vi "Get AccessType.vi"(8 "error in (no error)":errorcluster, 11 "PDO Mapping in":refnum<class "PDO Mapping.lvclass">) -> (0 "error out":errorcluster, 2 "AccessType":T1, 3 "PDO Mapping out":refnum<class "PDO Mapping.lvclass">)   [LabVIEW 2020, in "CANopen.lvlib" / "PDO Mapping.lvclass"]
uses:
  PDO Mapping.lvclass
  PDO Mapping.lvclass/PDO Mapping.ctl
  Typedefs/Access Type.ctl
  CANopen.lvlib
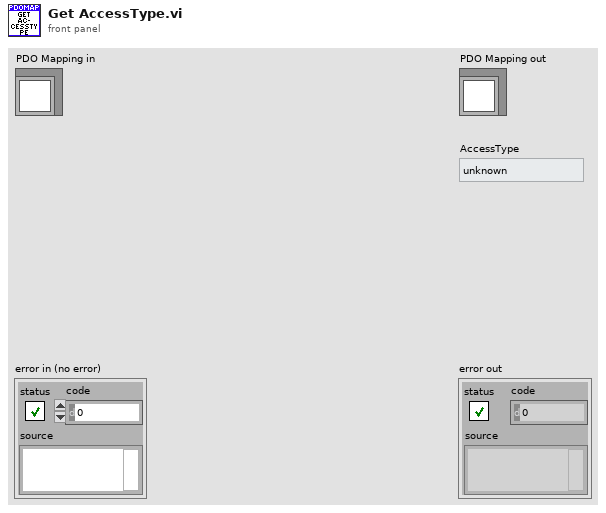
[diagram p1: front panel]
types:
  T1 = typedef "CANopen.lvlib/Access Type.ctl" = enum16{"unknown", "ro", "wo", "rw", "rwr", "rww", "const"}
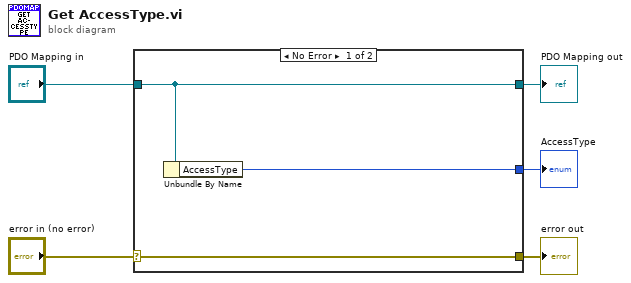
[diagram p0: block diagram]
diagram:
  n1 = case shown="No Error" "error in (no error)" {
    selector: "error in (no error)" -> [w8 w9]
    tunnel: [w8 w9] -> w4
    tunnel: [w7 w10] -> w2
    tunnel: "PDO Mapping in" -> [w7 w10]
    tunnel: [w6 _] -> w1
    frame No Error {
      n2 = Unbundle By Name(w7) -> ("AccessType"=w6:T1)
    }
    frame Error {
    }
  }
  "error out" <- w4
  "PDO Mapping out" <- w2
  "AccessType" <- w1
